vi "Insert Step.vi"(10 "Insert Above?":bool, 11 "Settings UI in":refnum<class "Settings UI.lvclass">) -> (3 "Settings UI out":refnum<class "Settings UI.lvclass">)   [LabVIEW 2020, in "Output Sequencer.lvlib" / "Settings UI.lvclass"]
uses:
  Settings UI.lvclass
  Settings UI.lvclass/Settings UI.ctl
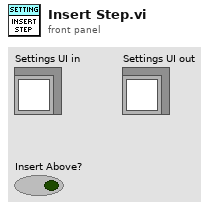
[diagram p1: front panel]
types:
  T1 = typedef "Output Sequencer.lvlib/Settings UI.lvclass/Step Settings.ctl" = cluster{"Description":string, "Precondition":string, "Duration":dbl, "Mode":string, "Delay Between Values":dbl, "Analog Values":string[], "Digital Values":string[], "Postcondition":string, "On True":string, "On False":string}
  T2 = cluster{"Left Cell String":string, "Child Text":string[], "Child Tag":string, "Item Indent":i32, "Child Only?":bool, "Glyph Index":i32}[]
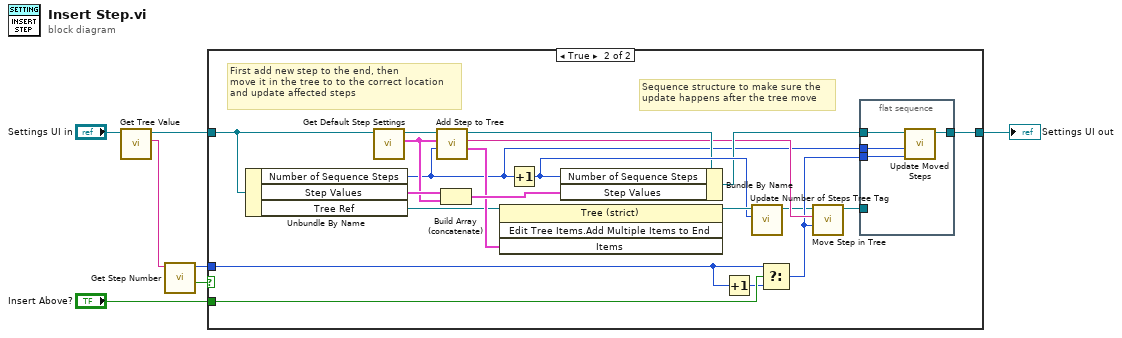
[diagram p0: block diagram]
diagram:
  n1 = call "Get Tree Value.vi"("UI Data in"="Settings UI in") -> ("Value"=w1:string, "UI Data out"=w6:refnum<class "Settings UI.lvclass">)  [unwired: 9 in]
  n2 = call "Get Step Number.vi"("Tree Tag"=w1) -> ("Is Step tag?"=w2:bool, "Step Number"=w3:i32)  [unwired: 8 in, 1 out]
  n3 = case shown="True" w2 {
    tunnel: w3 -> [_ w23]
    tunnel: w6 -> [w8 w11]
    tunnel: [w8 w17] -> w7
    tunnel: "Insert Above?" -> [_ w24]
    frame False {
    }
    frame True {
      # "Sequence structure to make sure the\nupdate happens after the tree move"
      # "First add new step to the end, then\nmove it in the tree to to the correct location\nand update affected steps"
      n4 = Unbundle By Name(w11) -> ("Number of Sequence Steps"=w9:i32, "Step Values"=w28:T1[], "Tree Ref"=w10:refnum<vi>)
      n5 = call "Get Default Step Settings.vi"("UI Data In"=w11) -> ("Default Step Settings"=w21:T1, "UI Data out"=w19:refnum<class "Settings UI.lvclass">)  [unwired: 9 in]
      n6 = call "Add Step to Tree.vi"("Step Index"=w9, "Step Settings"=w21, "UI Data In"=w19) -> ("Tree Items"=w20:T2, "Step tag"=w14:string, "UI Data out"=w18:refnum<class "Settings UI.lvclass">)  [unwired: 6 in]
      n7 = Build Array (concatenate)(w28, w21) -> (w27:T1[])
      n8 = invoke class="Tree (strict)" method="Edit Tree Items.Add Multiple Items to End"(reference=w10, "Items"=w20) -> (reference out=w26:refnum<vi>)  [unwired: 2 in, 3 out]
      n9 = Increment(x=w9) -> (x+1=w25:i32)
      n10 = Bundle By Name(cluster=w18, "Number of Sequence Steps"=w25, "Step Values"=w27) -> (w16:refnum<class "Settings UI.lvclass">)
      n11 = Increment(x=w23) -> (x+1=w22:i32)
      n12 = call "Update Number of Steps Tree Tag.vi"("New Number of Steps"=w25, "TreeControl in"=w26) -> ("TreeControl out"=w12:refnum<vi>)  [unwired: 9 in]
      n13 = Select(t=w23, s=w24, f=w22) -> (s? t:f=w13:i32)
      n14 = call "Move Step in Tree.vi"("New Position"=w13, "Step Tag"=w14, "TreeControl in"=w12) -> ("TreeControl out"=w15:refnum<vi>)  [unwired: 8 in]
      n15 = flat-sequence {
        tunnel: w9 -> [w32]
        tunnel: w13 -> [w31]
        tunnel: [w30] -> w17
        tunnel: w16 -> [w29]
        tunnel: w15 -> [_]
        frame #0 {
          n16 = call "Update Moved Steps.vi"("New Step Number"=w31, "Previous Step Number"=w32, "UI Data In"=w29) -> ("UI Data Out"=w30:refnum<class "Settings UI.lvclass">)  [unwired: 8 in]
        }
      }
    }
  }
  "Settings UI out" <- w7
